vi "GetOSBitness.vi"(8 "error in (no error)":errorcluster) -> (0 "error out":errorcluster, 2 "64-bit system":bool)   [LabVIEW 2022 SP3, in "MES_Local.lvlib" / "MES_Local.lvclass"]
uses:
  MES_Local.lvclass
panel:
  out "32-bit system":bool
  out "CMD Output":string="This is the output from Windows Command Prompt. "
  out "String before \"-bit\"":string="This the same output, but only the portion before \"-bit\" in the original output. "
  out "32/64 subset":string="Substring containing \"32\" or \"64\""
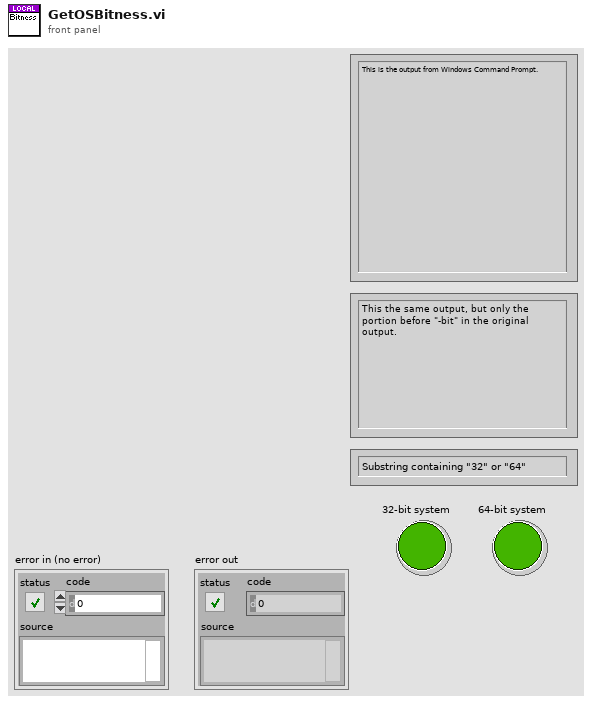
[diagram p1: front panel]
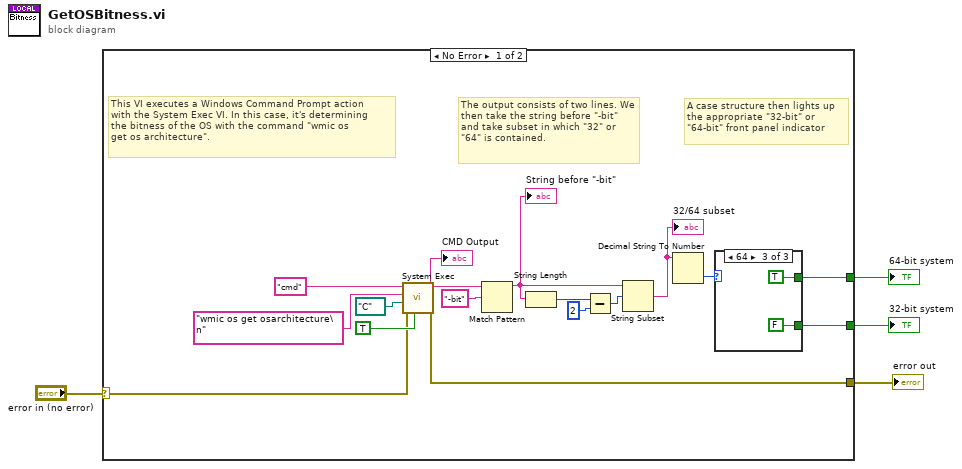
[diagram p0: block diagram]
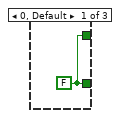
[diagram p2: hidden frame]
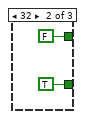
[diagram p3: hidden frame]
diagram:
  n1 = case shown="No Error" "error in (no error)" {
    selector: "error in (no error)" -> [w5 _]
    tunnel: [w8 _] -> w4
    tunnel: [w7 _] -> w3
    tunnel: [w6 _] -> w2
    frame No Error {
      # "A case structure then lights up\nthe appropriate \"32-bit\" or\n\"64-bit\" front panel indicator"
      # "The output consists of two lines. We then take the string before \"-bit\" and take subset in which \"32\" or \"64\" is contained."
      # "This VI executes a Windows Command Prompt action\nwith the System Exec VI. In this case, it's determining \nthe bitness of the OS with the command \"wmic os \nget os architecture\"."
      n2 = call <vilib>:"System Exec.vi"("run minimized? (F)"=TRUE, "error in (no error)"=w5, "working directory"=path "C:/", "standard input"="wmic os get osarchitecture\n", "command line"="cmd") -> ("error out"=w6:errorcluster, "standard output"=w9:string)  [unwired: 3 in, 2 out]
      "CMD Output" <- w9
      n3 = Match Pattern(string=w9, regular expression="-bit") -> (before substring=w10:string)  [unwired: 1 in, 3 out]
      "String before \"-bit\"" <- w10
      n4 = String Length(string=w10) -> (length=w15:i32)
      n5 = Subtract(x=w15, y=2) -> (x-y=w13:i32)
      n6 = String Subset(string=w10, offset (0)=w13) -> (substring=w11:string)  [unwired: 1 in]
      "32/64 subset" <- w11
      n7 = Decimal String To Number(string=w11) -> (number=w12:i32)  [unwired: 2 in, 1 out]
      n8 = case shown="64" w12 {
        tunnel: [w21 FALSE TRUE] -> w8
        tunnel: [w21 TRUE FALSE] -> w7
        frame 0, Default {
          w21 = FALSE
        }
        frame 32 {
        }
        frame 64 {
        }
      }
    }
    frame Error {
    }
  }
  "32-bit system" <- w3
  "64-bit system" <- w4
  "error out" <- w2
